vi "Do.vi"(8 "error in (no error)":errorcluster, 10 "Actor in":refnum<class "Actor.lvclass">, 11 "Update PV":refnum<class "Update-PV Msg.lvclass">) -> (0 "error out":errorcluster, 2 "Actor out":refnum<class "Actor.lvclass">)   [LabVIEW 2014, in "CS++GUIActor.lvlib" / "Update-PV Msg.lvclass"]
doc: "(<B>Filename</B>: Actor Framework.lvlib:Message.lvclass:Do.vi)\n\nDefines what a message does when it is received by an actor. Generally, a message instructs an actor to invoke one of its methods.\n\nBy default, this method does nothing. A child class must override it to define behavior. Create a child class by using the Actor Framework Message Maker dialog box."
uses:
  Update-PV Msg.lvclass
  <vilib>/ActorFramework/Actor/Actor.lvclass
  CS++GUIActor/CS++GUIActor.lvclass
  CS++PVMonitor Messages/CS++PVUpdate Msg/CS++PVUpdate Msg.lvclass/CS++PVUpdate Msg.ctl
  Classes/CS++ProcessVariables/ProcessVariable/PV.lvclass
  CS++PVMonitor Messages/CS++PVUpdate Msg/CS++PVUpdate Msg.lvclass
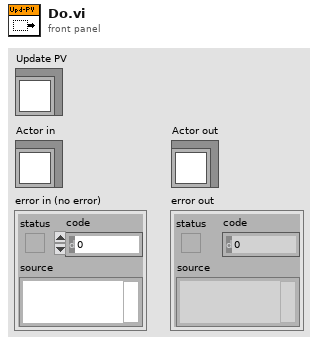
[diagram p1: front panel]
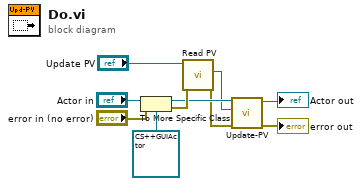
[diagram p0: block diagram]
diagram:
  n1 = To More Specific Class(target class=refnum<class "CS++GUIActor.lvclass"> refnum ("CS++GUIActor.lvlib:CS++GUIActor.lvclass"), reference="Actor in", error in="error in (no error)") -> (specific class reference=w6:refnum<class "CS++GUIActor.lvclass">, error out=w7:errorcluster)
  n2 = call "Read PV.vi"("error in (no error)"=w7, "CS++PVUpdate Msg in"="Update PV") -> ("error out"=w4:errorcluster, "PV"=w5:refnum<class "PV.lvclass">)  [unwired: 7 in, 1 out]
  n3 = call "Update-PV.vi"("Error In"=w4, "PV"=w5, "CS++GUIActor in"=w6) -> ("Error Out"=→"error out":errorcluster, "CS++GUIActor out"=→"Actor out":refnum<class "CS++GUIActor.lvclass">)  [unwired: 7 in]
